vi "Y0M Traceability.vi"(0 "HW_Config":string[][](array[string]), 1 "Barcode":string, 2 "Data Cluster":T1, 3 "Part no":string, 4 "station_Name":string, 5 "SEQ_Config":T5(array[cluster]), 6 "Test List":refnum<vi>, 7 "Model/Variant":T4, 8 "Shift":string, 9 "SEQ Name":string, 11 "error in (no error)":errorcluster, 12 "Step No":i32) -> (10 "Data Cluster out":T1, 15 "error out":errorcluster)   [LabVIEW 2017]
uses:
  controls/Auto UI Data.ctl
  controls/Configuration Details.ctl
  IPC/MQTT/Q Driver/Controls/IPC-MQTT-Q driver-Q Options.ctl
  IPC/MQTT/Controls/Publish data.ctl
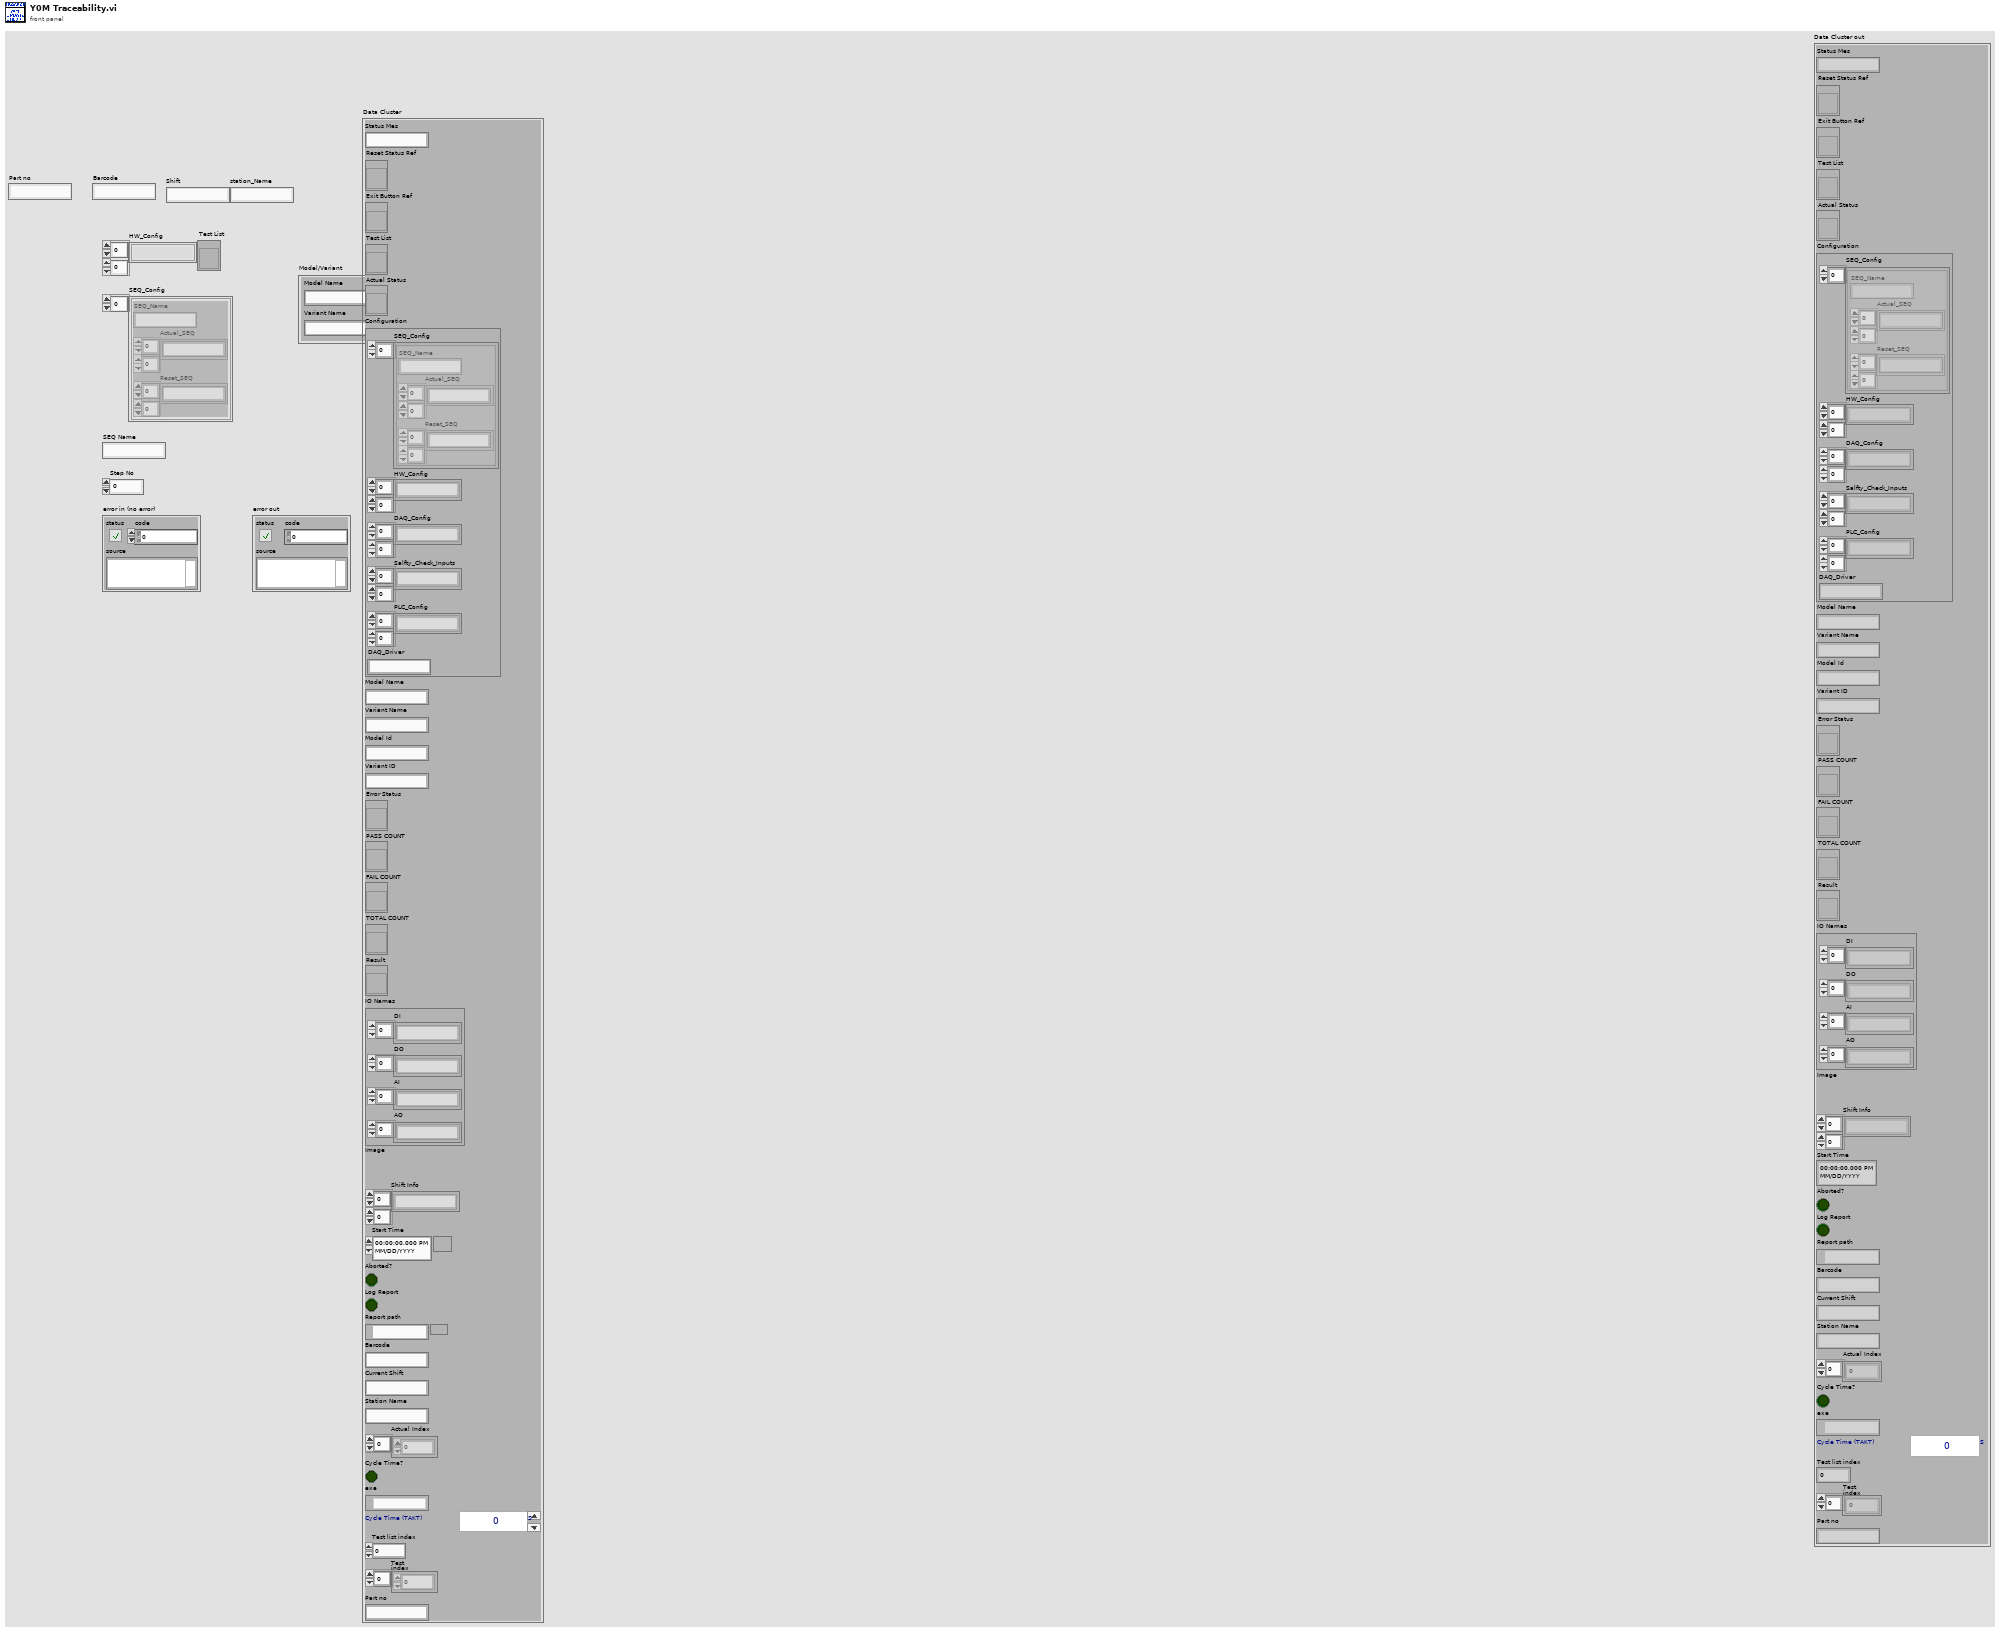
[diagram p1: front panel]
types:
  T1 = typedef "Auto UI Data.ctl" = cluster{"Status Mes":string, "Reset Status Ref":refnum<vi>, "Exit Button Ref":refnum<vi>, "Test List":refnum<vi>, "Actual Status":refnum<vi>, "Configuration":T2, "Model Name":string, "Variant Name":string, "Model Id":string, "Variant ID":string, "Error Status":refnum<vi>, "PASS COUNT":refnum<vi>, "FAIL COUNT":refnum<vi>, "TOTAL COUNT":refnum<vi>, "Result":refnum<vi>, "IO Names":cluster{"DI":string[], "DO":string[], "AI":string[], "AO":string[]}, "Image":T3, "Shift Info":string[][], "Start Time":timestamp, "Aborted?":bool, "Log Report":bool, "Report path":path, "Barcode":string, "Current Shift":string, "Station Name":string, "Actual Index":i32[], "Cycle Time?":bool, "exe":path, "Cycle Time (TAKT)":u16, "Test list index":u32, "Test index":u32[], "Part no":string}
  T2 = typedef "Configuration Details.ctl" = cluster{"SEQ_Config":cluster{"SEQ_Name":string, "Actual_SEQ":string[][], "Reset_SEQ":string[][]}[], "HW_Config":string[][], "DAQ_Config":string[][], "Salfty_Check_Inputs":string[][], "PLC_Config":string[][], "DAQ_Driver":string}
  T3 = typedef "IMAQ Image.ctl" = refnum<image>
  T4 = cluster{"Model Name":string, "Variant Name":string}
  T5 = cluster{"SEQ_Name":string, "Actual_SEQ":string[][], "Reset_SEQ":string[][]}[]
  T6 = typedef "Publish data.ctl" = cluster{"Topic":string, "Message":string}
  T7 = typedef "IPC-MQTT-Q driver-Q Options.ctl" = enum16{"En Q", "En Q N", "De Q", "Init", "En Q N Stack", "Flush", "Close"}
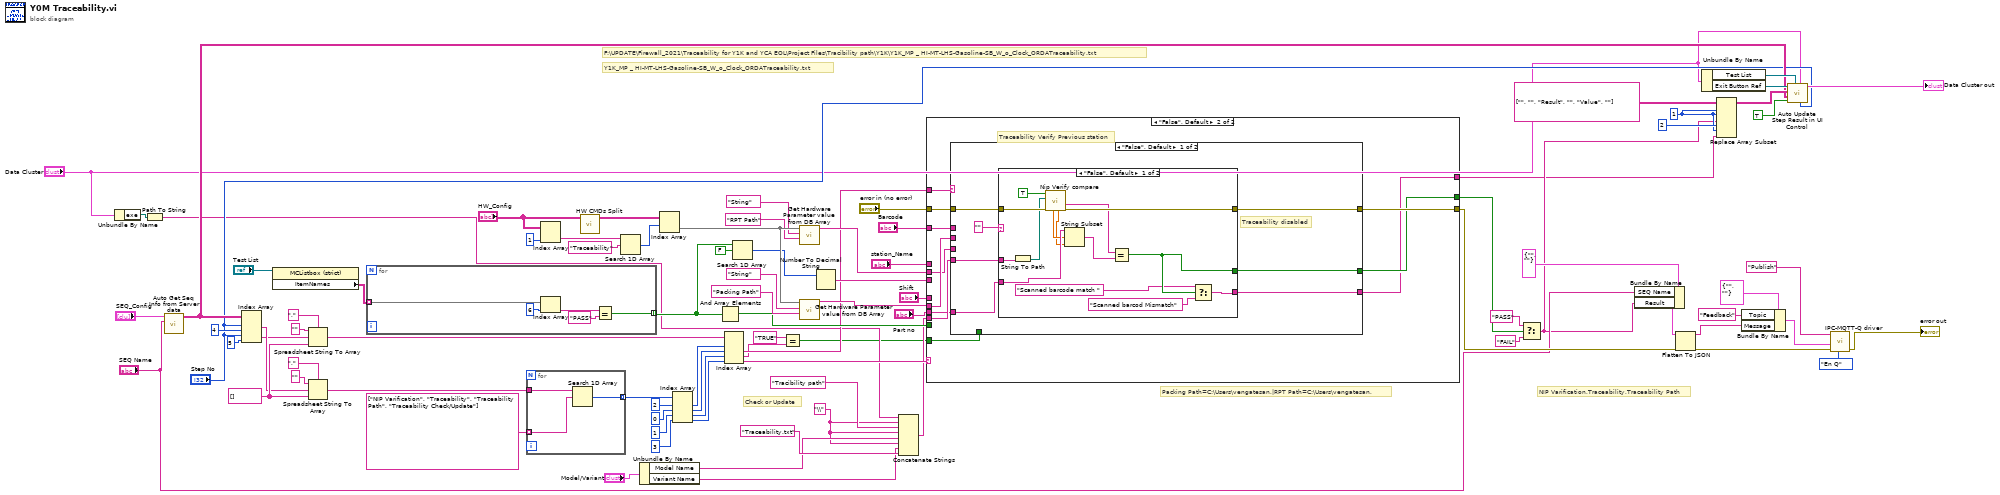
[diagram p0: block diagram]
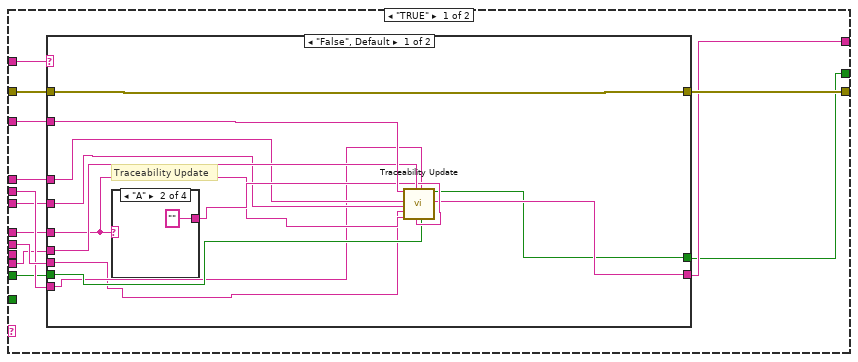
[diagram p2: hidden frame]
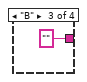
[diagram p4: hidden frame]
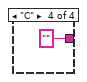
[diagram p5: hidden frame]
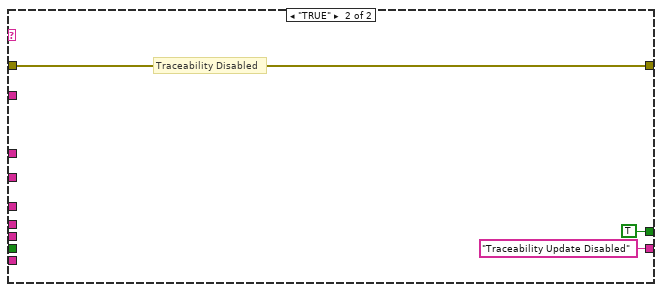
[diagram p6: hidden frame]
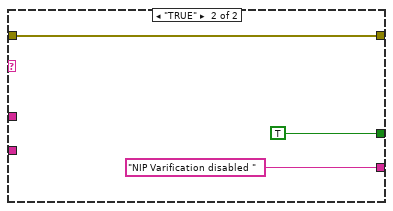
[diagram p7: hidden frame]
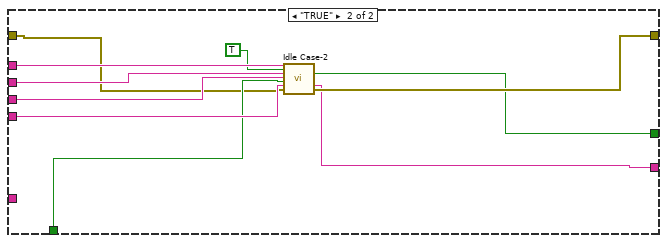
[diagram p8: hidden frame]
diagram:
  w16 = 1 ("index (row)")
  w5 = "\\" ("string")
  w75 = string[] []
  # "F:\\UPDATE\\Firewall_2021\\Traceability for Y1K and YCA EOL\\Project Files\\Tracibility path\\Y1K\\Y1K_MP _ HI-MT-LHS-Gasoline-SB_W_o_Clock_ORDATraceability.txt"
  # "Y1K_MP _ HI-MT-LHS-Gasoline-SB_W_o_Clock_ORDATraceability.txt"
  # "Check or Update"
  # "NIP Varification,Traceability,Traceability Path"
  # "Packing Path=C:\\Users\\vengatesan,|RPT Path=C:\\Users\\vengatesan,"
  n1 = Unbundle By Name("Data Cluster") -> ("exe"=w9:path)
  n2 = Path To String(path=w9) -> (string=w8:string)
  n3 = call "Auto Get Seq Info from Server data.vi"("SEQ Name"="SEQ Name", "SEQ_Config"="SEQ_Config") -> ("Reset_SEQ"=w13:string[][])  [unwired: 8 in, 1 out]
  n4 = Index Array(array=w13, index (row) #1="Step No", index (col) #1=4 ("disabled index (col)"), index (row) #2="Step No", index (col) #2=5 ("disabled index (col)")) -> (element #1=w74:string, element #2=w73:string)
  n5 = property class="MCListbox (strict)"(reference="Test List") -> ("ItemNames"=w49:string[][])  [unwired: 1 in, 2 out]
  n6 = Spreadsheet String To Array(delimiter (Tab)=",", format string="", spreadsheet string=w73, array type (2D Dbl)=w75) -> (array=w78:string[])
  n7 = Spreadsheet String To Array(delimiter (Tab)=",", format string="", spreadsheet string=w74, array type (2D Dbl)=w75) -> (array=w76:string[])
  n8 = for {
    tunnel: w49 -> [w94] mode=indexing
    tunnel: [w90] -> w45 mode=indexing
    n9 = Index Array(array=w94, index=6) -> (element=w92:string)
    n10 = Equal?(x=w92, y="PASS") -> (x = y?=w90:bool)
  }
  n11 = for {
    tunnel: w76 -> [w97]
    tunnel: string[] ["NIP Varification", "Traceability", "Traceability Path", "Traceability Check/Update"] -> [w96] mode=indexing
    tunnel: [w95] -> w79 mode=indexing
    n12 = Search 1D Array(1D array=w97, element=w96) -> (index of element=w95:i32)  [unwired: 1 in]
  }
  n13 = Index Array(array="HW_Config", index (col)=1 ("disabled index (col)")) -> (element=w56:string[])  [unwired: 1 in]
  n14 = call "HW CMDs Split.vi"("queryresult"="HW_Config") -> ("Array"=w59:string[][])  [unwired: 10 in]
  n15 = Search 1D Array(1D array=w56, element="Traceability") -> (index of element=w60:i32)  [unwired: 1 in]
  n16 = Unbundle By Name("Model/Variant") -> ("Model Name"=w7:string, "Variant Name"=w6:string)
  n17 = Index Array(array=w59, index (row)=w60) -> (element=w65:string[])  [unwired: 1 in]
  n18 = Index Array(array=w79, index #1=2 ("index"), index #2=0 ("index"), index #3=1 ("index"), index #4=3 ("index")) -> (element #1=w83:i32, element #2=w85:i32, element #3=w86:i32, element #4=w88:i32)
  n19 = And Array Elements(Boolean array=w45) -> (logical AND=w44:bool)
  n20 = Index Array(array=w78, index #1=w83, index #2=w85, index #3=w86, index #4=w88) -> (element #2=w42:string, element #3=w4:string, element #4=w89:string)  [unwired: 1 out]
  n21 = Search 1D Array(1D array=w45, element=FALSE) -> (index of element=w47:i32)  [unwired: 1 in]
  n22 = Equal?(x="TRUE", y=w4) -> (x = y?=w2:bool)
  n23 = call "Get Hardware Parameter value from DB Array.vi"("Parameter Name"="RPT Path", "Data Type"="String", "Data"=w65) -> ("String"=w68:string)  [unwired: 4 in, 4 out]
  n24 = call "Get Hardware Parameter value from DB Array.vi"("Parameter Name"="Packing Path", "Data Type"="String", "Data"=w65) -> ("String"=w67:string)  [unwired: 4 in, 4 out]
  n25 = Number To Decimal String(number=w47) -> (decimal integer string=w46:string)  [unwired: 1 in]
  n26 = Concatenate Strings(w8, w5, "Tracibility path" ("string"), w5, w7, w5, w6, "Traceability.txt" ("string")) -> (w39:string)
  n27 = case shown="\"False\", Default" w89 {
    tunnel: "Barcode" -> [w110 w139]
    tunnel: w67 -> [w109 w138]
    tunnel: w68 -> [w108 w137]
    tunnel: w39 -> [w107 w136]
    tunnel: "error in (no error)" -> [w106 w135]
    tunnel: [w105 w134] -> w29
    tunnel: w42 -> [w104 w133]
    tunnel: "Shift" -> [w103 _]
    tunnel: w46 -> [w102 _]
    tunnel: w44 -> [w101 _]
    tunnel: "station_Name" -> [w100 _]
    tunnel: [w98 w132] -> w26
    tunnel: [w99 w131] -> w14
    tunnel: w2 -> [_ w130]
    tunnel: "Part no" -> [_ w129]
    frame "TRUE" {
      n28 = case shown="\"False\", Default" w104 {
        tunnel: w110 -> [w122 _]
        tunnel: w109 -> [w111 _]
        tunnel: w108 -> [w112 _]
        tunnel: w107 -> [w121 _]
        tunnel: w106 -> [w115 w128]
        tunnel: [w115 w128] -> w105
        tunnel: w103 -> [w119 _]
        tunnel: w102 -> [w118 _]
        tunnel: w101 -> [w117 _]
        tunnel: w100 -> [w116 _]
        tunnel: [w114 "Traceability Update Disabled" ("messageOut")] -> w99
        tunnel: [w113 TRUE ("updated_successfully_status")] -> w98
        frame "False", Default {
          # "Traceability Update"
          n29 = case shown="\"A\"" w119 {
            tunnel: [_ "" "" ""] -> w120
            frame Default {
            }
            frame "A" {
            }
            frame "B" {
            }
            frame "C" {
            }
          }
          n30 = call "Traceability Update.vi"("Barcode"=w122, "Station_Name"=w116, "Error_Code"=w118, "PackgingPath"=w111, "Shift"=w119, "Traceability_File_Path"=w121, "OperatorID"=w120, "RPTPath"=w112, "Result"=w117) -> ("updated_successfully?"=w113:bool, "MessageOut"=w114:string)  [unwired: 8 in, 1 out]
        }
        frame "TRUE" {
          # "Traceability Disabled"
        }
      }
    }
    frame "False", Default {
      # "Traceability Verify Previous station"
      n31 = case shown="\"False\", Default" w133 {
        tunnel: w139 -> [_ w173]
        tunnel: w138 -> [_ w172]
        tunnel: w137 -> [_ w171]
        tunnel: w136 -> [w144 w170]
        tunnel: w135 -> [w146 w164]
        tunnel: [w145 w169] -> w134
        tunnel: [w142 w168] -> w132
        tunnel: [w140 w167] -> w131
        tunnel: w130 -> [_ w166]
        tunnel: w129 -> [w141 _]
        frame "False", Default {
          # "Traceability disabled"
          n32 = case shown="\"False\", Default" "" {
            tunnel: w146 -> [w160 w163]
            tunnel: [w159 w163] -> w145
            tunnel: w144 -> [w158 _]
            tunnel: [w156 TRUE ("verified")] -> w142
            tunnel: w141 -> [w151 _]
            tunnel: [w154 "NIP Varification disabled " ("messageOut")] -> w140
            frame "False", Default {
              n33 = String To Path(string=w158) -> (path=w157:path)
              n34 = call "Nip Verify compare.vi"("error in"=w160, "file path (use dialog)"=w157, "NIP Enable/Disable"=TRUE) -> ("error out"=w159:errorcluster, "LCD Part No"=w152:string, "Part no Length"=w148:dbl, "Part no Offset"=w149:dbl)  [unwired: 3 in, 2 out]
              n35 = String Subset(string=w151, offset (0)=w149, length (rest)=w148) -> (substring=w150:string)
              n36 = Equal?(x=w152, y=w150) -> (x = y?=w156:bool)
              n37 = Select(t="Scanned barcode match ", s=w156, f="Scanned barcod Mismatch") -> (s? t:f=w154:string)
            }
            frame "TRUE" {
            }
          }
        }
        frame "TRUE" {
          n38 = call "Idle Case-2.vi"("Barcode"=w173, "NIP Verification"=TRUE, "Packing Path"=w172, "RPT Path"=w171, "Traceability"=w166, "Traceabilityfilepath"=w170, "error in"=w164) -> ("Verified?"=w168:bool, "MessageOut"=w167:string, "error out"=w169:errorcluster)  [unwired: 17 in, 1 out]
        }
      }
    }
  }
  n39 = Select(t="PASS" ("Message"), s=w26, f="FAIL" ("Message")) -> (s? t:f=w15:string)
  n40 = Bundle By Name(cluster=cluster{"SEQ Name":string, "Result":string} {"SEQ Name"="", "Result"=""} ("Client FB"), "SEQ Name"="SEQ Name", "Result"=w15) -> (w31:cluster{"SEQ Name":string, "Result":string})
  n41 = Flatten To JSON(anything=w31, error in (no error)=w29) -> (JSON string=w30:string, 11:w32:errorcluster)  [unwired: 1 in]
  n42 = Unbundle By Name("Data Cluster") -> ("Test List"=w19:refnum<vi>, "Exit Button Ref"=w22:refnum<vi>)
  n43 = Replace Array Subset(array=string[][] [["", ""], ["Result", ""], ["Value", ""]] ("Step Result"), new element #1=w15, index (row) #1=w16, index (col) #1=w16, new element #2=w14, index (row) #2=2 ("index (row)"), index (col) #2=w16) -> (w18:string[][])
  n44 = Bundle By Name(cluster=T6 {"Topic"="", "Message"=""} ("Cluster"), "Topic"="Feedback", "Message"=w30) -> (w34:T6)
  n45 = call "Auto Update Step Result in UI Control.vi"("Step No"="Step No", "Data Cluster in"="Data Cluster", "Test List"=w19, "Acutal(T)/Reset(F)?"=TRUE, "Reset_SEQ"=w13, "Step Result"=w18, "Boolean in"=w22) -> ("Data Cluster out"=→"Data Cluster out":T1)  [unwired: 4 in]
  n46 = call "IPC-MQTT-Q driver.vi"("Q Options"=IPC-MQTT-Q_driver-Q_Options."En Q", "error in (no error)"=w32, "Message Data"=w34, "Message"="Publish") -> ("error out"=→"error out":errorcluster)  [unwired: 5 in, 2 out]
